vi "SerialPort.Auto Find Port.vi"(4 "PID":string, 6 "VID":string, 8 "error in (no error)":errorcluster, 11 "SerialPort in":refnum<class "SerialPort.lvclass">) -> (0 "error out":errorcluster, 2 "VISA resource name":refnum<visa-resource-name>, 3 "SerialPort out":refnum<class "SerialPort.lvclass">)   [LabVIEW 2018, in "SerialPort.lvclass"]
uses:
  SerialPort.lvclass
  Controls/SerialPort.Status Enum.ctl
  SerialPort.lvclass/SerialPort.ctl
  Utils/Errors/Error.Error Code List.ctl
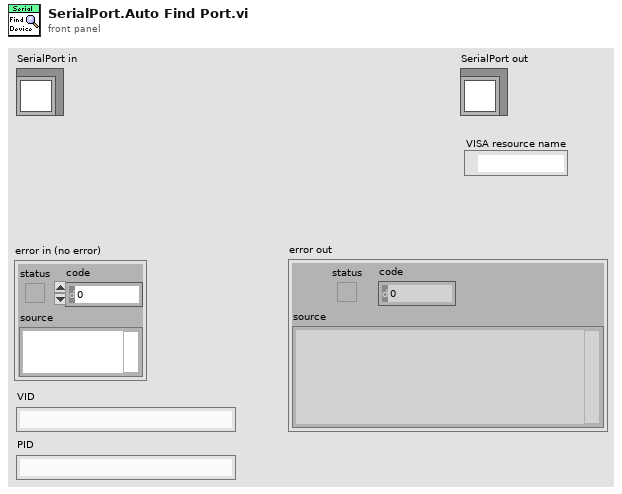
[diagram p1: front panel]
types:
  T1 = typedef "SerialPort.Status Enum.ctl" = enum16{"Disconnected", "Connecting", "Connected"}
  T2 = typedef "Error.Error Code List.ctl" = i32
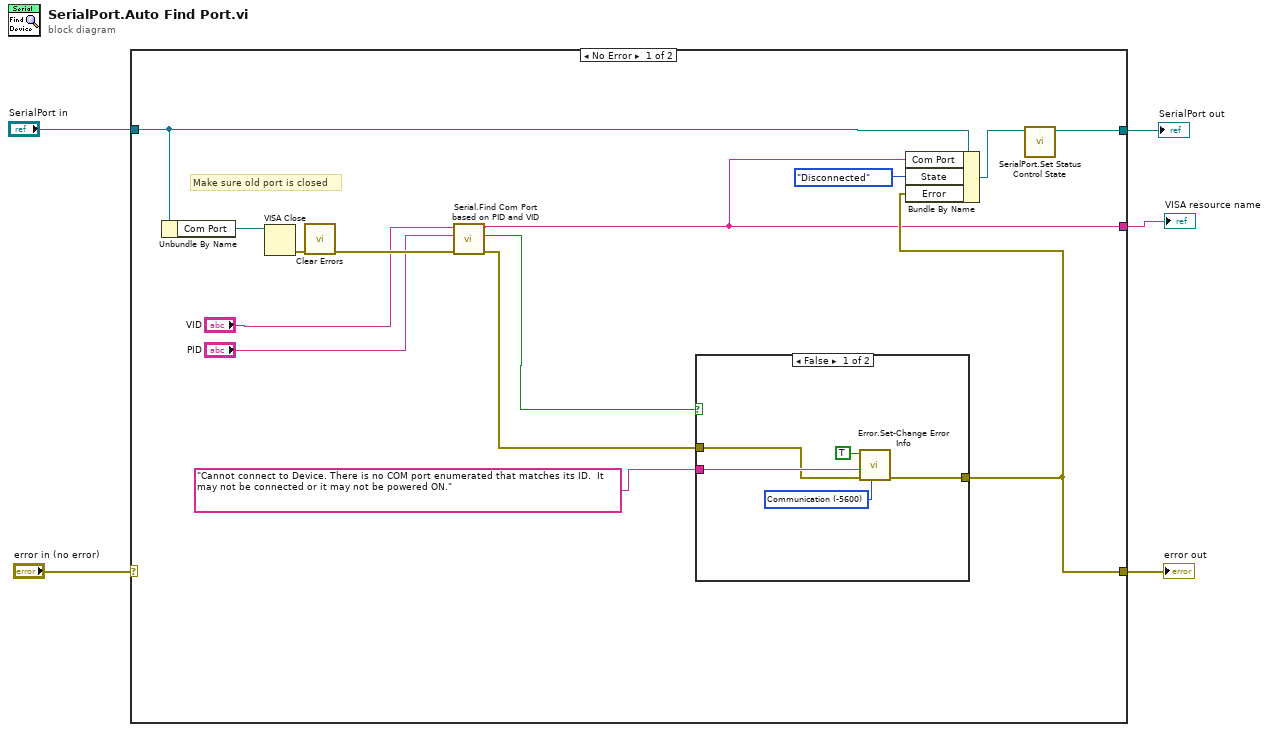
[diagram p0: block diagram]
diagram:
  n1 = case shown="No Error" "error in (no error)" {
    selector: "error in (no error)" -> [_ w26]
    tunnel: [w14 w26] -> w4
    tunnel: [w19 w25] -> w2
    tunnel: "SerialPort in" -> [w13 w25]
    tunnel: [w8 _] -> w1
    frame No Error {
      # "Make sure old port is closed"
      n2 = Unbundle By Name(w13) -> ("Com Port"=w16:refnum<visa-resource-name>)
      n3 = VISA Close(VISA resource name=w16) -> (error out=w17:errorcluster)  [unwired: 1 in]
      n4 = call <vilib>:"Clear Errors.vi"("error in (no error)"=w17) -> ("error out"=w12:errorcluster)  [unwired: 5 in, 1 out]
      n5 = call "Serial.Find Com Port based on PID and VID.vi"("error in"=w12, "PID"="PID", "VID"="VID") -> ("error out"=w7:errorcluster, "Found"=w9:bool, "COM Port"=w8:string)  [unwired: 4 in, 2 out]
      n6 = case shown="False" w9 {
        tunnel: [w20 _] -> w14
        tunnel: w7 -> [w21 _]
        tunnel: "Cannot connect to Device. There is no COM port enumerated that matches its ID.  It may not be connected or it may not be powered ON." ("source") -> [w22 _]
        frame False {
          w24 = T2 -5600 items=["No Error"=0, "Abort"=-2, "Misc"=-5000, "Fixture Error"=-5100, "File IO - General"=-5200, "FIle IO - Config Error"=-5201, "Instrument - General"=-5300, "Instrument - Serial Com"=-5301, "Instrument - Camera"=-5302, "Instrument - PS"=-5303, "Instrument - Oscilloscope"=-5304, "Instrument - Function Gen"=-5305, "Instrument - Load"=-5306, "Instrument - Meter"=-5307, "Instrument - Power Control"=-5308, "Instrument - Motion"=-5309, "Instrument - RF"=-5310, "System Exe"=-5400, "Image Processing"=-5500, "Communication"=-5600, "Script - Syntax Error"=-6000, "Script - Invalid Name or Param"=-6100, "Script - Timeout"=-6200, "Invalid Data"=-6300] ("Std Code")
          n7 = call "Error.Set-Change Error Info.vi"("Std Code"=w24, "error in"=w21, "Description"=w22, "Set Error"=TRUE) -> ("error out"=w20:errorcluster)  [unwired: 7 in]
        }
        frame True {
        }
      }
      n8 = Bundle By Name(cluster=w13, "Com Port"=w8, "State"=SerialPort.Status_Enum."Disconnected", "Error"=w14) -> (w18:refnum<class "SerialPort.lvclass">)
      n9 = call "SerialPort.Set Status Control State.vi"("SerialPort in"=w18) -> ("SerialPort out"=w19:refnum<class "SerialPort.lvclass">)  [unwired: 9 in, 1 out]
    }
    frame Error {
    }
  }
  "error out" <- w4
  "SerialPort out" <- w2
  "VISA resource name" <- w1
